vi "TestExecutive.vi"() -> ()   [LabVIEW 2025]
uses:
  controls/TestDefinition.ctl
  controls/TestType.ctl
  controls/TestExecStates.ctl
  <vilib>/Utility/error.llb/DialogType.ctl
  <vilib>/Utility/error.llb/Error Cluster From Error Code.vi
  <vilib>/ErrorRing/Error Ring.xnode
panel:
  out "Camera":string="USB Camera"
  out "TopFolderPath":path=path "E:/LTM Tests/HeaterTest_25-01-22_17-59-34"
  out "TopFolderPrefix":string="HeaterTest_25-01-22_17-59-34"
  in  "Server IP":u16(ring) items=["localhost", "172.17.52.10"]
  out "Status":string="Waiting for Rising trigger. Target = -50.000000"
  in  "Main Tabs":T1(tab)=enum."TestDefinition"
  in  "Next Button 2":bool
  in  "Loggers Directory":path=path "E:/LTM Tests/MechanismLTM"
  in  "Test Name":string="HeaterTest"
  in  "FFMPEG exe":path=path "C:/Program Files/FFMpeg/bin/ffmpeg.exe"
  in  "Path to Actuation Script":path=path "C:/Users/Public/Documents/ob_egse-ABU_LTM_MotorTesting/egse.py"
  in  "StartCycle":i32
  in  "Next Button":bool
  in  "PSU_Monitor":waveform(dbl)[](array[waveform])=[{"t0"=timestamp(3820413812.1099424 s since 1904-01-01), "dt"=1.0, "Y"=[2.52], "attributes"=variant("NI_ChannelName"=variant(string "Board_Voltage_0"))}, {"t0"=timestamp(3820413812.1153584 s since 1904-01-01), "dt"=1.0, "Y"=[-0.009], "attributes"=variant("NI_ChannelName"=variant(string "Board_Voltage_0"))}, {"t0"=timestamp(3820413812.1099424 s since 1904-01-01), "dt"=1.0, "Y"=[-0.017], "attributes"=variant("NI_ChannelName"=variant(string "Board_Current_0"))}, {"t0"=timestamp(3820413812.1153584 s since 1904-01-01), "dt"=1.0, "Y"=[0.0], "attributes"=variant("NI_ChannelName"=variant(string "Board_Current_0"))}]
  in  "Heater Monitor":waveform(dbl)[](array[waveform])=[{"t0"=timestamp(3820413812.092942 s since 1904-01-01), "dt"=1.0, "Y"=[-0.005], "attributes"=variant("NI_ChannelName"=variant(string "Heater_Voltage"))}, {"t0"=timestamp(3820413812.092942 s since 1904-01-01), "dt"=1.0, "Y"=[-0.002], "attributes"=variant("NI_ChannelName"=variant(string "Heater_Current"))}]
  in  "Video Camera":u16(ring) items=["USB Camera"]
  out "ChannelNames":string[](array[string])=["3A", "3B", "3C", "3D", "4A", "4B", "4C", "4D", "Target"]
  in  "ControlChannel":u16(ring) items=["3A", "3B", "3C", "3D", "4A", "4B", "4C", "4D", "Target"]
  in  "TVC_Temperatures":waveform(dbl)[](array[waveform])=[{"t0"=timestamp(3820413812.1049423 s since 1904-01-01), "dt"=1.0, "Y"=[-80.0], "attributes"=variant("NI_ChannelName"=variant(string "3A"))}, {"t0"=timestamp(3820413812.1049423 s since 1904-01-01), "dt"=1.0, "Y"=[0.1969585335155295], "attributes"=variant("NI_ChannelName"=variant(string "3B"))}, {"t0"=timestamp(3820413812.1049423 s since 1904-01-01), "dt"=1.0, "Y"=[0.2898606356704896], "attributes"=variant("NI_ChannelName"=variant(string "3C"))}, {"t0"=timestamp(3820413812.1049423 s since 1904-01-01), "dt"=1.0, "Y"=[0.3274623555028864], "attributes"=variant("NI_ChannelName"=variant(string "3D"))}, {"t0"=timestamp(3820413812.1049423 s since 1904-01-01), "dt"=1.0, "Y"=[0.3794250746071903], "attributes"=variant("NI_ChannelName"=variant(string "4A"))}, {"t0"=timestamp(3820413812.1049423 s since 1904-01-01), "dt"=1.0, "Y"=[0.7650917242886434], "attributes"=variant("NI_ChannelName"=variant(string "4B"))}, {"t0"=timestamp(3820413812.1049423 s since 1904-01-01), "dt"=1.0, "Y"=[0.4416685188806395], "attributes"=variant("NI_ChannelName"=variant(string "4C"))}, {"t0"=timestamp(3820413812.1049423 s since 1904-01-01), "dt"=1.0, "Y"=[0.7497510727682433], "attributes"=variant("NI_ChannelName"=variant(string "4D"))}, {"t0"=timestamp(3820413812.1049423 s since 1904-01-01), "dt"=1.0, "Y"=[0.8015992709050663], "attributes"=variant("NI_ChannelName"=variant(string "Target"))}]
  in  "TLUP_Temperatures":waveform(dbl)[](array[waveform])=[{"t0"=timestamp(3820413812.102944 s since 1904-01-01), "dt"=1.0, "Y"=[23.56152], "attributes"=variant("NI_ChannelName"=variant(string "TLUP_0"))}, {"t0"=timestamp(3820413812.102944 s since 1904-01-01), "dt"=1.0, "Y"=[-999.0], "attributes"=variant("NI_ChannelName"=variant(string "TLUP_1"))}, {"t0"=timestamp(3820413812.102944 s since 1904-01-01), "dt"=1.0, "Y"=[-999.0], "attributes"=variant("NI_ChannelName"=variant(string "TLUP_2"))}, {"t0"=timestamp(3820413812.102944 s since 1904-01-01), "dt"=1.0, "Y"=[-999.0], "attributes"=variant("NI_ChannelName"=variant(string "TLUP_3"))}, {"t0"=timestamp(3820413812.102944 s since 1904-01-01), "dt"=1.0, "Y"=[nan], "attributes"=variant("NI_ChannelName"=variant(string "TLUP_4"))}, {"t0"=timestamp(3820413812.102944 s since 1904-01-01), "dt"=1.0, "Y"=[nan], "attributes"=variant("NI_ChannelName"=variant(string "TLUP_5"))}, {"t0"=timestamp(3820413812.102944 s since 1904-01-01), "dt"=1.0, "Y"=[nan], "attributes"=variant("NI_ChannelName"=variant(string "TLUP_6"))}, {"t0"=timestamp(3820413812.102944 s since 1904-01-01), "dt"=1.0, "Y"=[nan], "attributes"=variant("NI_ChannelName"=variant(string "TLUP_7"))}]
  in  "PSU Enable":bool
  in  "Heater Enable":bool
  in  "COM Port":i32=21 min=1 max=63 step=1
  in  "TestDefinition":T2={"Tests"=[{"TTrigger"=-130.0, "Direction"=enum."Falling", "TDelay"=0.0, "Type"=enum."No Test", "Heater Test (s)"=0.0, "Pre-Log (s)"=0.0, "Post-Log(s)"=0.0}, {"TTrigger"=-80.0, "Direction"=enum."Rising", "TDelay"=0.0, "Type"=enum."Heater Test", "Heater Test (s)"=900.0, "Pre-Log (s)"=10.0, "Post-Log(s)"=100.0}, {"TTrigger"=-50.0, "Direction"=enum."Rising", "TDelay"=30.0, "Type"=enum."No Test", "Heater Test (s)"=0.0, "Pre-Log (s)"=0.0, "Post-Log(s)"=0.0}, {"TTrigger"=-50.0, "Direction"=enum."Rising", "TDelay"=0.0, "Type"=enum."Heater Test", "Heater Test (s)"=150.0, "Pre-Log (s)"=10.0, "Post-Log(s)"=0.0}, {"TTrigger"=-50.0, "Direction"=enum."Rising", "TDelay"=0.0, "Type"=enum."Actuation Test", "Heater Test (s)"=0.0, "Pre-Log (s)"=2.0, "Post-Log(s)"=10.0}, {"TTrigger"=-45.0, "Direction"=enum."Rising", "TDelay"=0.0, "Type"=enum."Actuation Test", "Heater Test (s)"=30.0, "Pre-Log (s)"=10.0, "Post-Log(s)"=100.0}, {"TTrigger"=-35.0, "Direction"=enum."Rising", "TDelay"=0.0, "Type"=enum."Actuation Test", "Heater Test (s)"=30.0, "Pre-Log (s)"=10.0, "Post-Log(s)"=100.0}, {"TTrigger"=-25.0, "Direction"=enum."Rising", "TDelay"=0.0, "Type"=enum."Actuation Test", "Heater Test (s)"=30.0, "Pre-Log (s)"=10.0, "Post-Log(s)"=100.0}, {"TTrigger"=-15.0, "Direction"=enum."Rising", "TDelay"=0.0, "Type"=enum."Actuation Test", "Heater Test (s)"=30.0, "Pre-Log (s)"=10.0, "Post-Log(s)"=100.0}, {"TTrigger"=0.0, "Direction"=enum."Rising", "TDelay"=0.0, "Type"=enum."Actuation Test", "Heater Test (s)"=30.0, "Pre-Log (s)"=10.0, "Post-Log(s)"=100.0}, {"TTrigger"=10.0, "Direction"=enum."Rising", "TDelay"=0.0, "Type"=enum."Actuation Test", "Heater Test (s)"=30.0, "Pre-Log (s)"=10.0, "Post-Log(s)"=100.0}, {"TTrigger"=30.0, "Direction"=enum."Rising", "TDelay"=0.0, "Type"=enum."Actuation Test", "Heater Test (s)"=30.0, "Pre-Log (s)"=10.0, "Post-Log(s)"=100.0}, {"TTrigger"=40.0, "Direction"=enum."Rising", "TDelay"=0.0, "Type"=enum."Actuation Test", "Heater Test (s)"=30.0, "Pre-Log (s)"=10.0, "Post-Log(s)"=100.0}, {"TTrigger"=40.0, "Direction"=enum."Rising", "TDelay"=30.0, "Type"=enum."No Test", "Heater Test (s)"=30.0, "Pre-Log (s)"=10.0, "Post-Log(s)"=100.0}], "ActuationsPerLoop"=2, "Temperature\nLog Period(ms)"=1000, "PSU \nLog Period (ms)"=100} {"Tests"."Post-Log(s)" format="%#_13g"; "Tests"."Pre-Log (s)" format="%#_13g"; "Tests"."Heater Test (s)" format="%#_13g"}
  in  "Next Button 3":bool
  out "Master Logging":bool=TRUE
  out "DelayRemaining":string="00:00"
  out "Heater On":bool
  out "Temperatures":dynamicdata(graph)
  out "Trigger Point Reading":dbl=-80.0
  out "Actuation Logging":bool
  out "Heater Logging":bool
  in  "CyclesRemaining":i32
  in  "TempCycleNo":i32
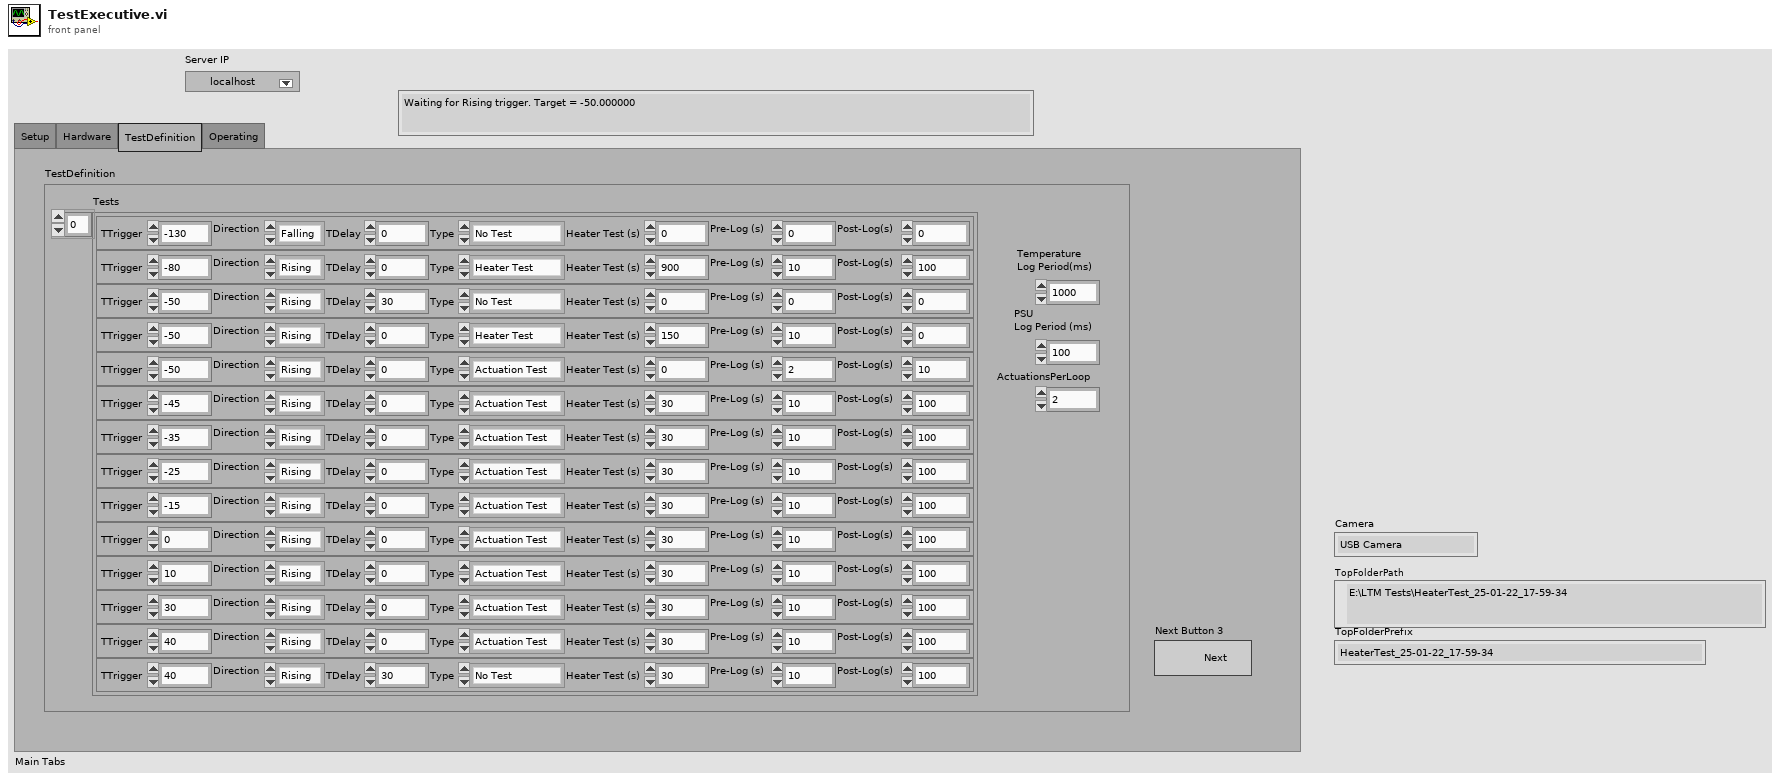
[diagram p1: front panel]
types:
  T1 = enum32{"Setup", "Hardware", "TestDefinition", "Operating"}
  T2 = typedef "TestDefinition.ctl" = cluster{"Tests":cluster{"TTrigger":dbl, "Direction":enum16{"Rising", "Falling"}, "TDelay":dbl, "Type":T3, "Heater Test (s)":dbl, "Pre-Log (s)":dbl, "Post-Log(s)":dbl}[], "ActuationsPerLoop":i32, "Temperature\nLog Period(ms)":i64, "PSU \nLog Period (ms)":i64}
  T3 = typedef "TestType.ctl" = enum16{"No Test", "Heater Test", "Actuation Test"}
  T4 = typedef "TestExecStates.ctl" = enum16{"Initialise", "Check Inputs", "Check Hardware", "Review Tests", "RunTests", "AbortExit", "Shutdown"}
  T5 = enum32{"Invalid Status", "Unconnected", "Active", "Idle", "Error", "Connecting"}
  T6 = typedef "LVDataSocketStatusTypeDef.ctl" = cluster{"Code":enum32{"Invalid Status", "Unconnected", "Active", "Idle", "Error", "Connecting"}, "Text":string}
  T7 = typedef "DialogType.ctl" = u16
  T8 = cluster{"TTrigger":dbl, "Direction":enum16{"Rising", "Falling"}, "TDelay":dbl, "Type":T3, "Heater Test (s)":dbl, "Pre-Log (s)":dbl, "Post-Log(s)":dbl}[]
  T9 = typedef "FFMpegRef.ctl" = cluster{"FFMpegRef":refnum<k24>, "StdOutRef":refnum<k24>, "DiagRef":refnum<k24>}
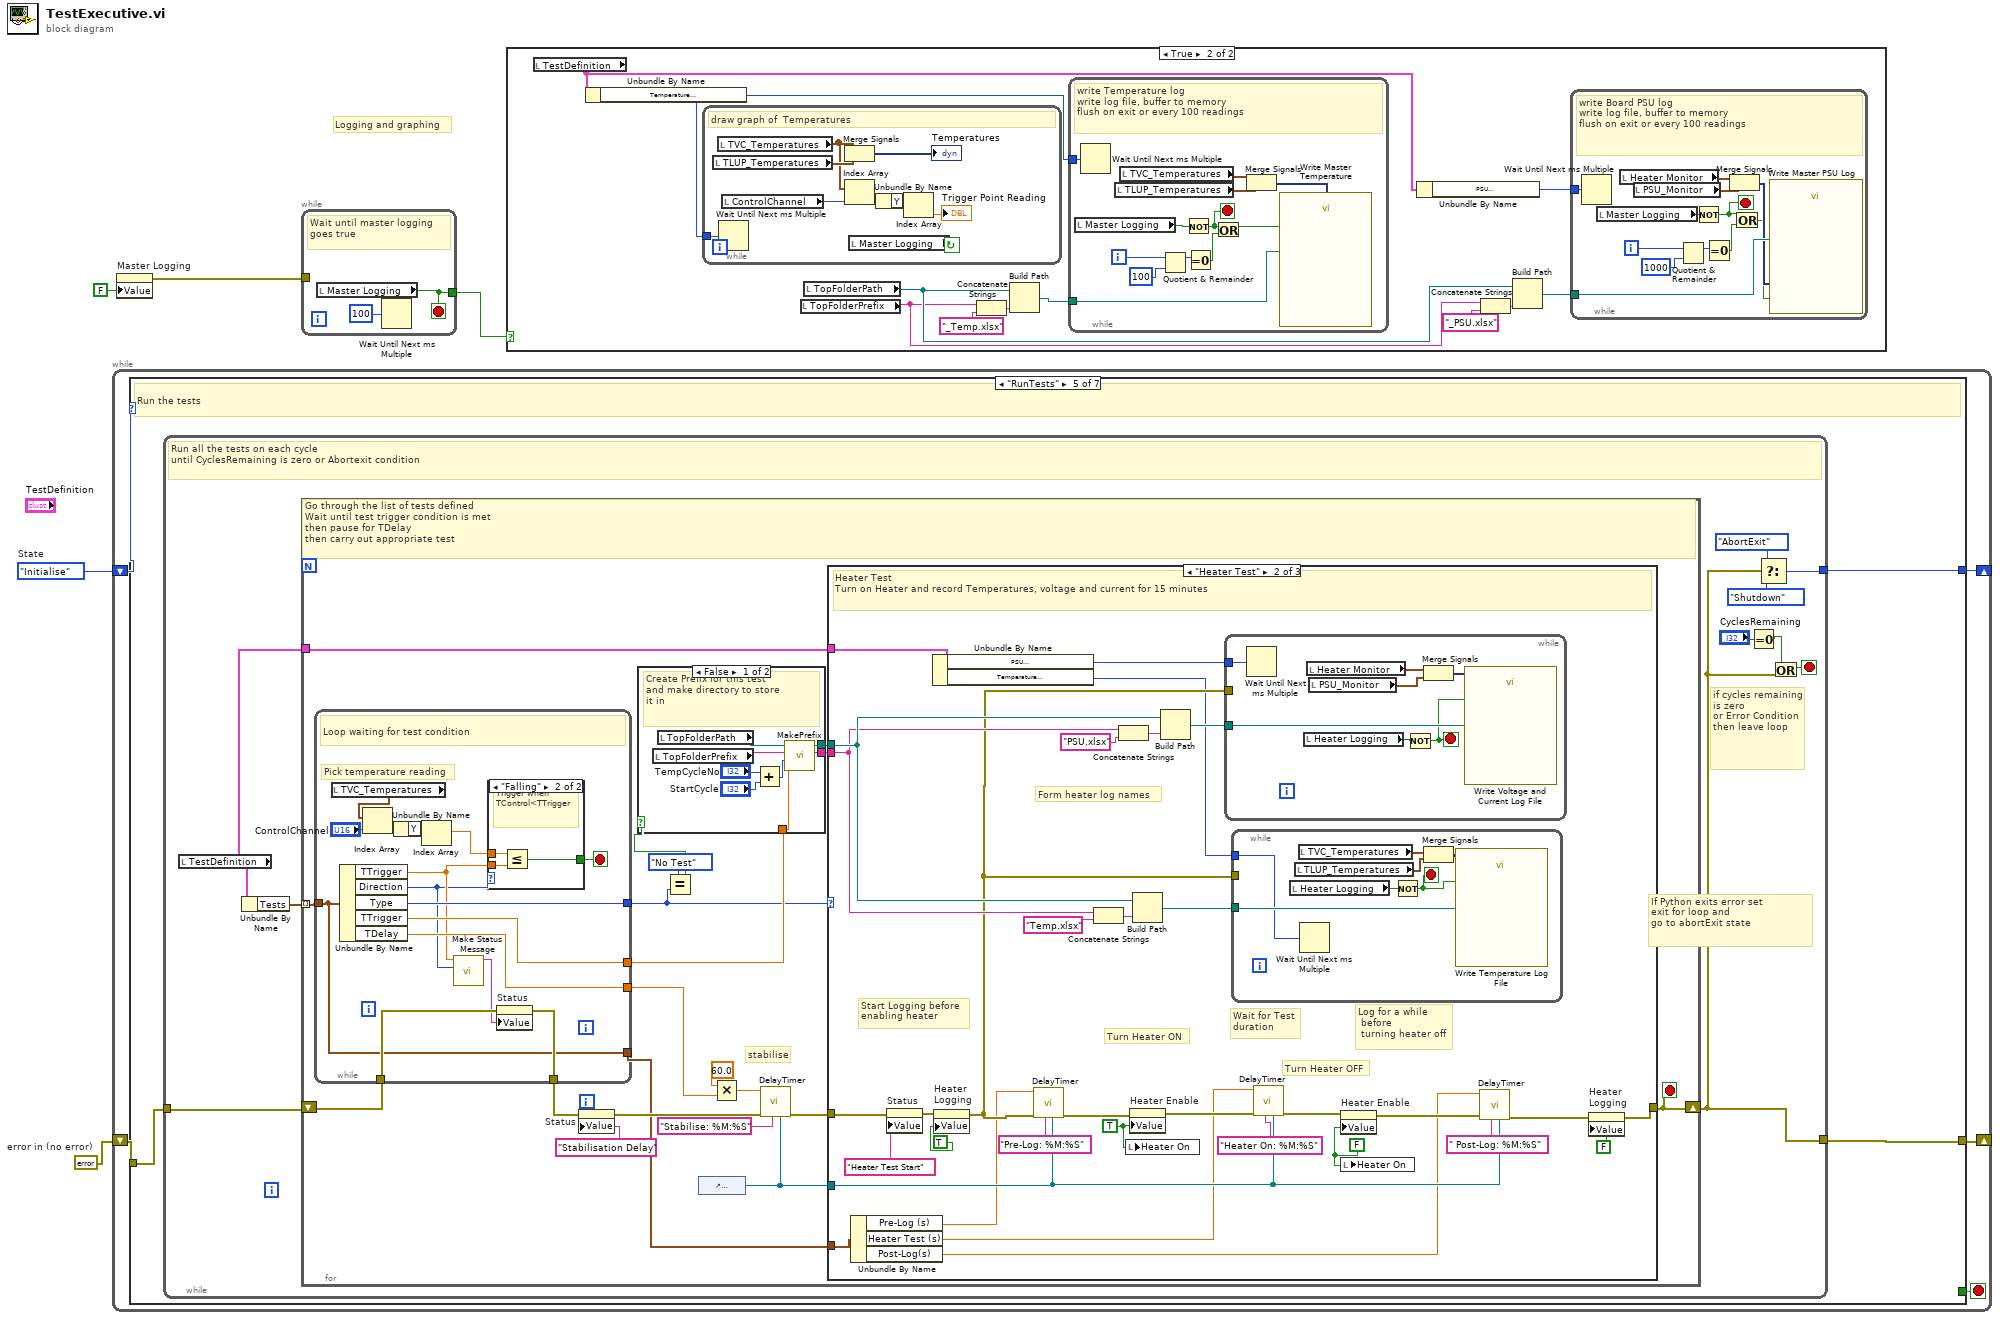
[diagram p0: block diagram]
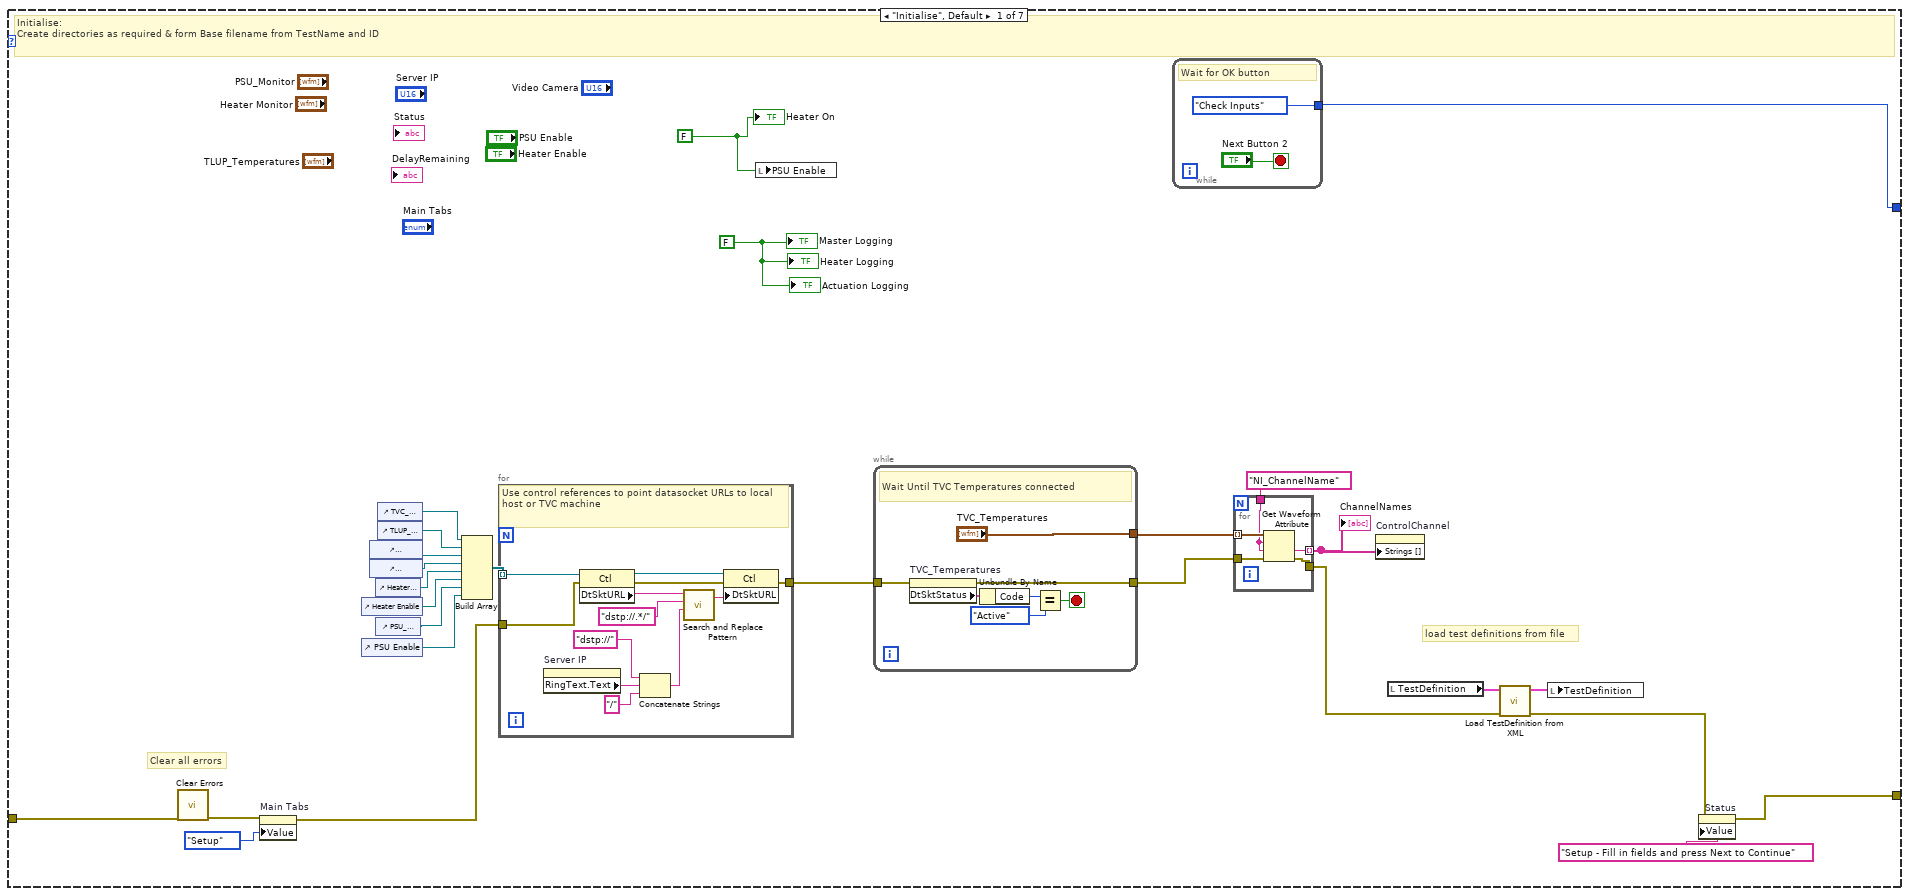
[diagram p3: hidden frame]
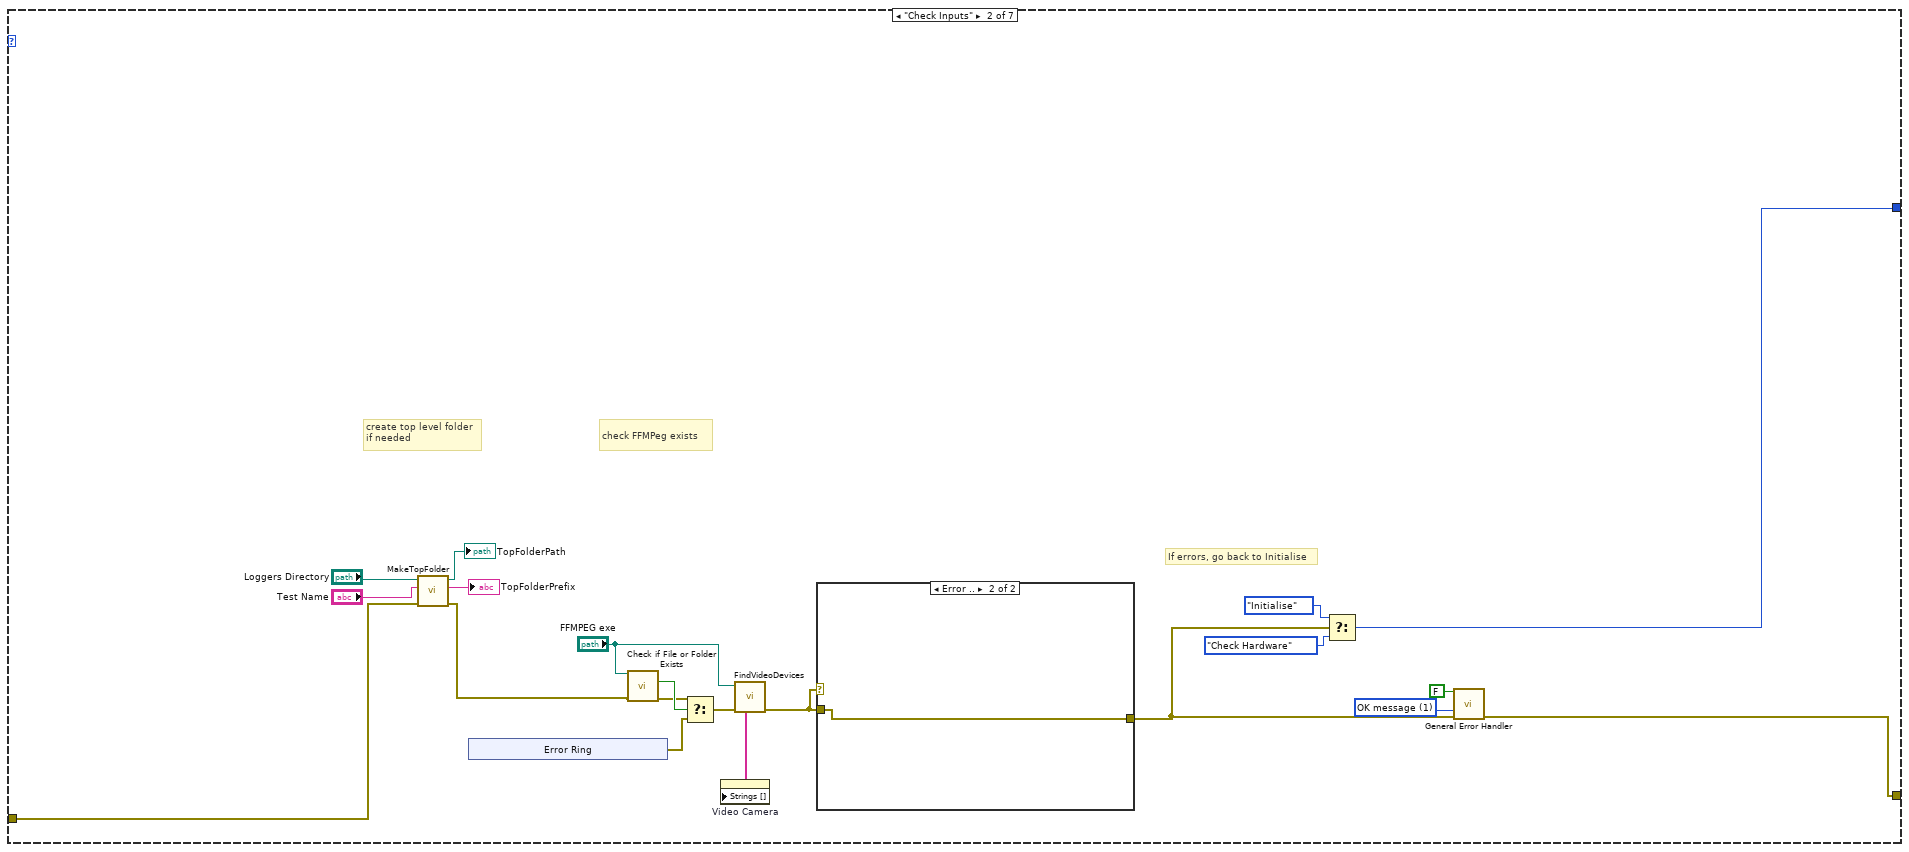
[diagram p4: hidden frame]
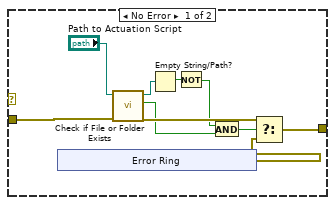
[diagram p5: hidden frame]
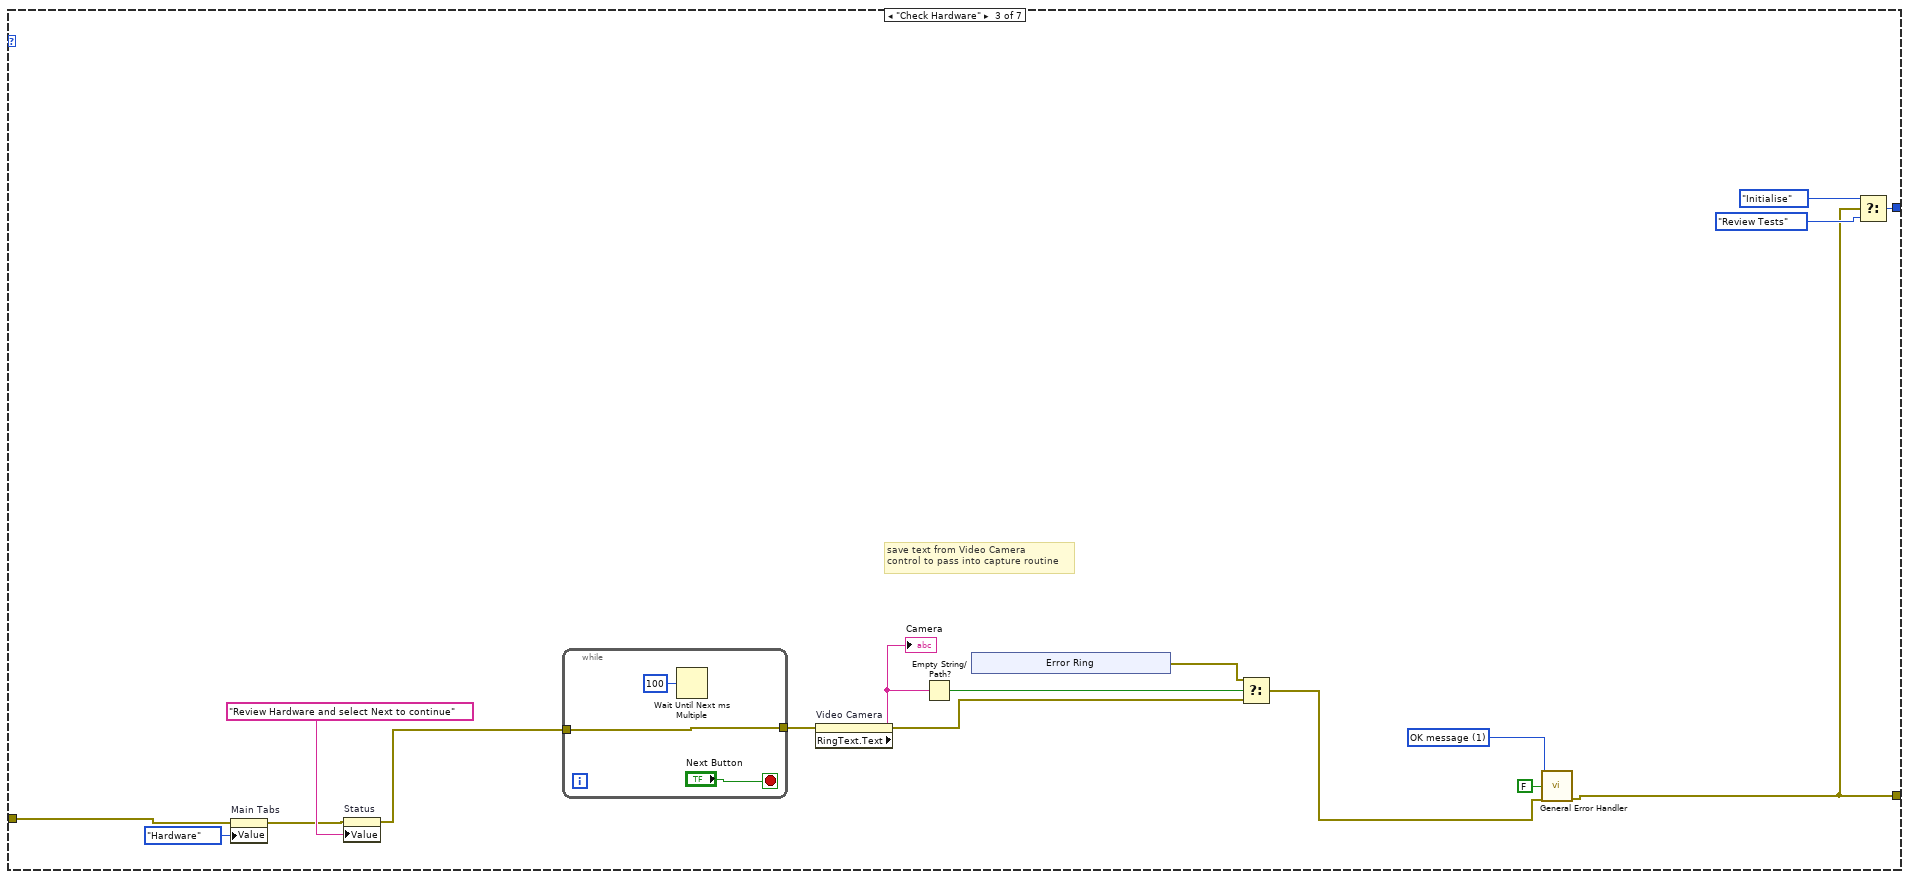
[diagram p6: hidden frame]
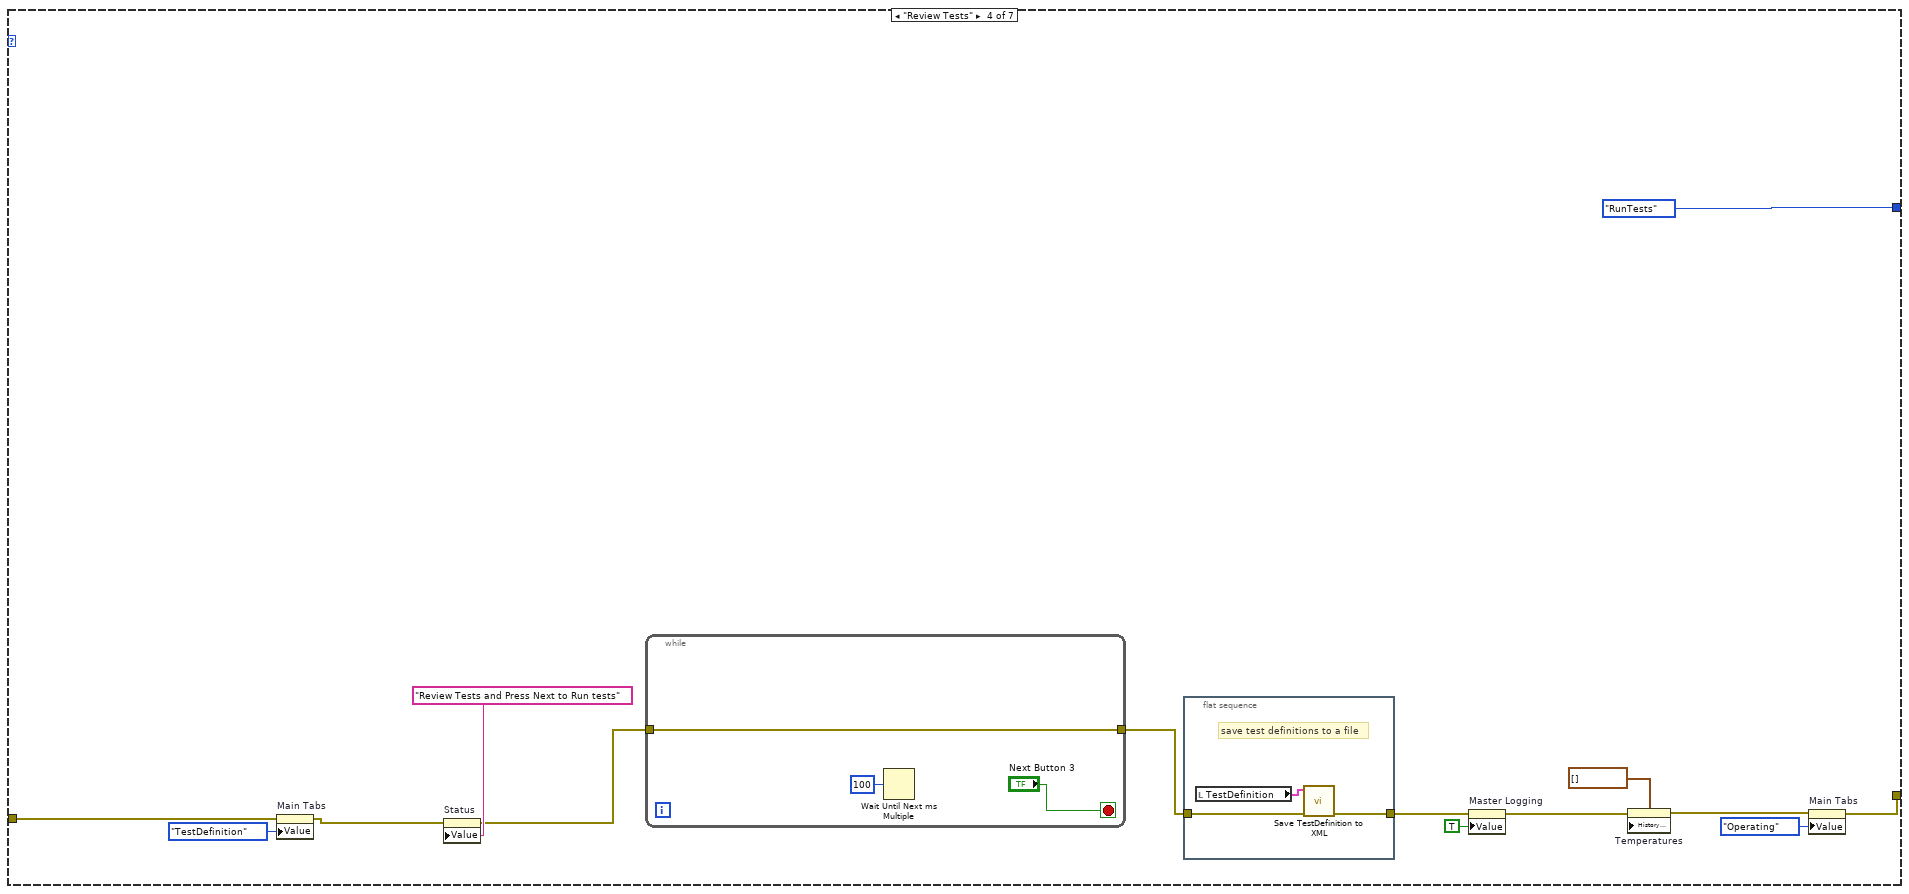
[diagram p7: hidden frame]
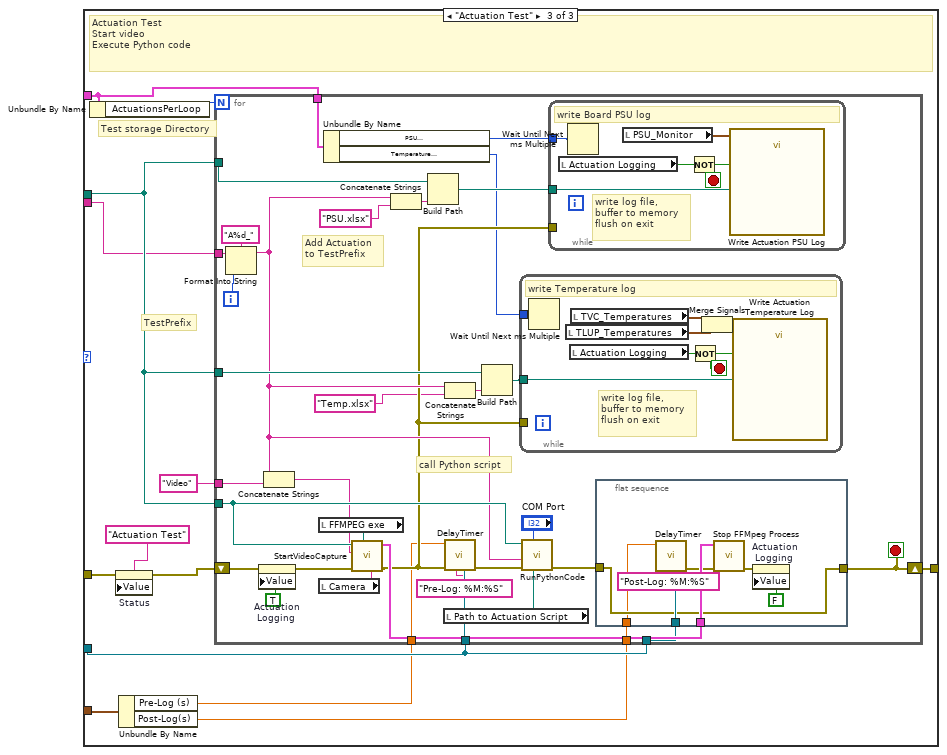
[diagram p10: hidden frame]
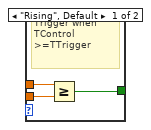
[diagram p11: hidden frame]
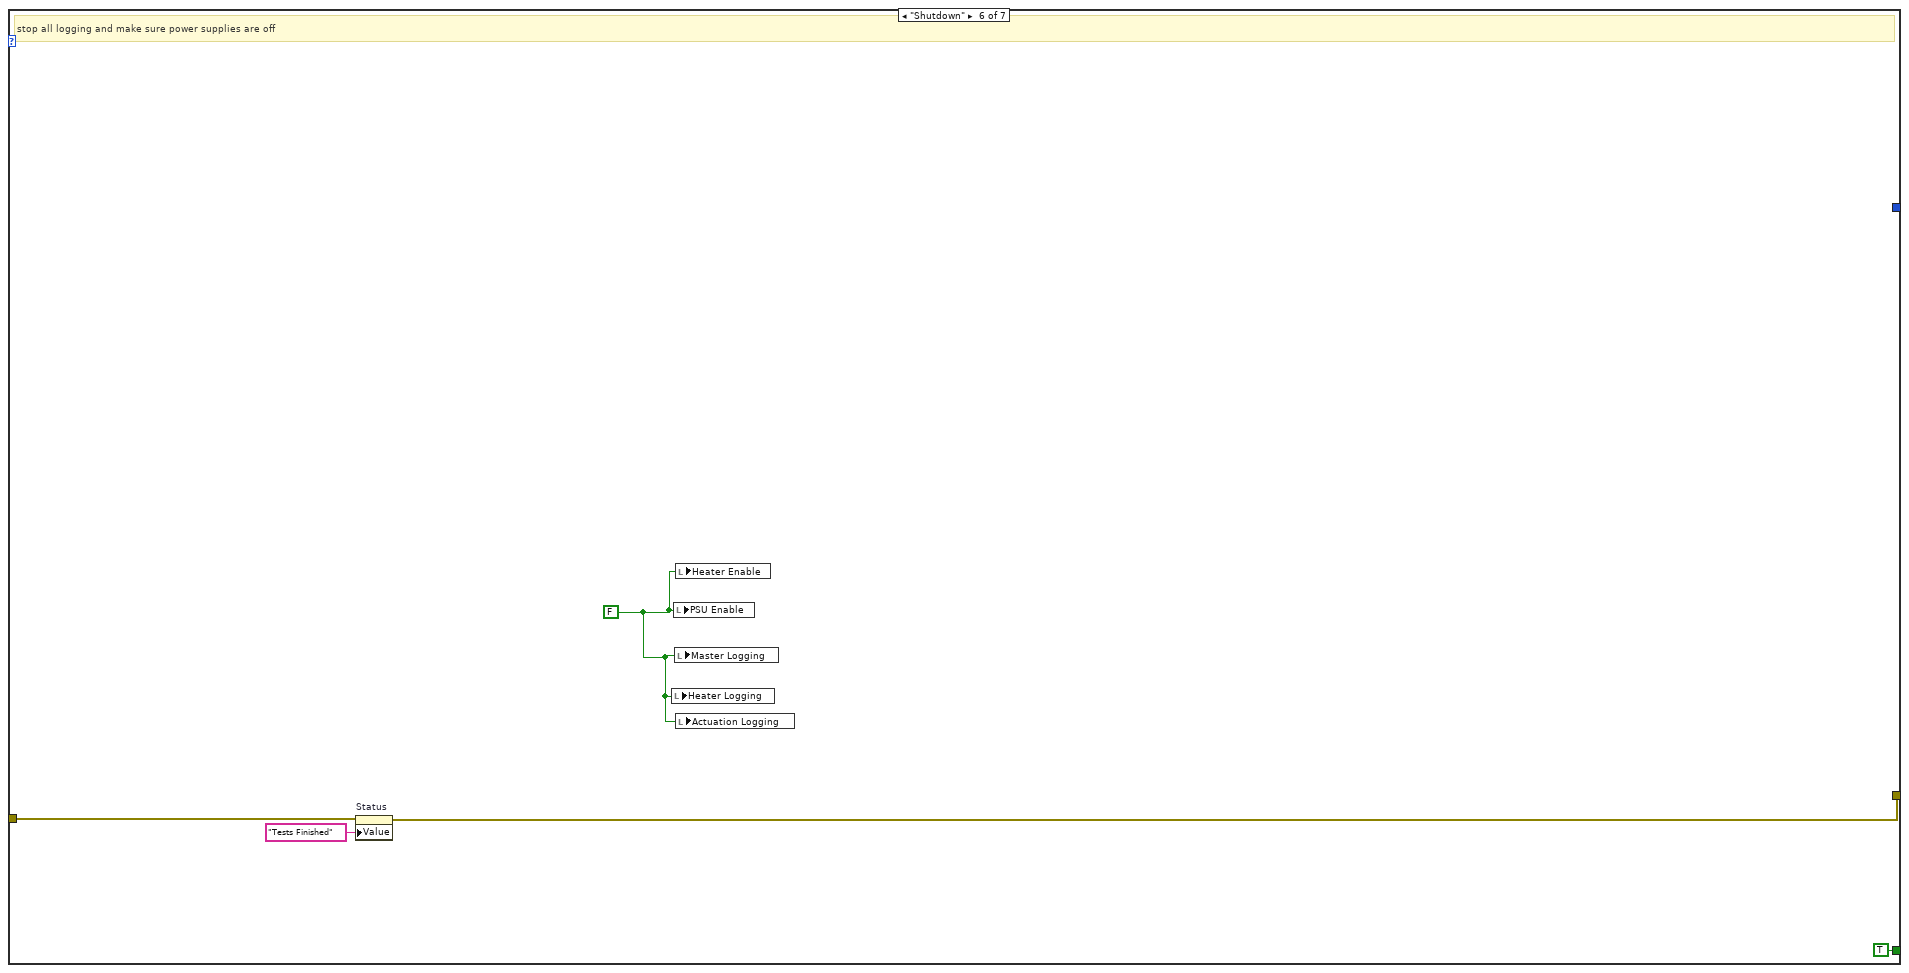
[diagram p12: hidden frame]
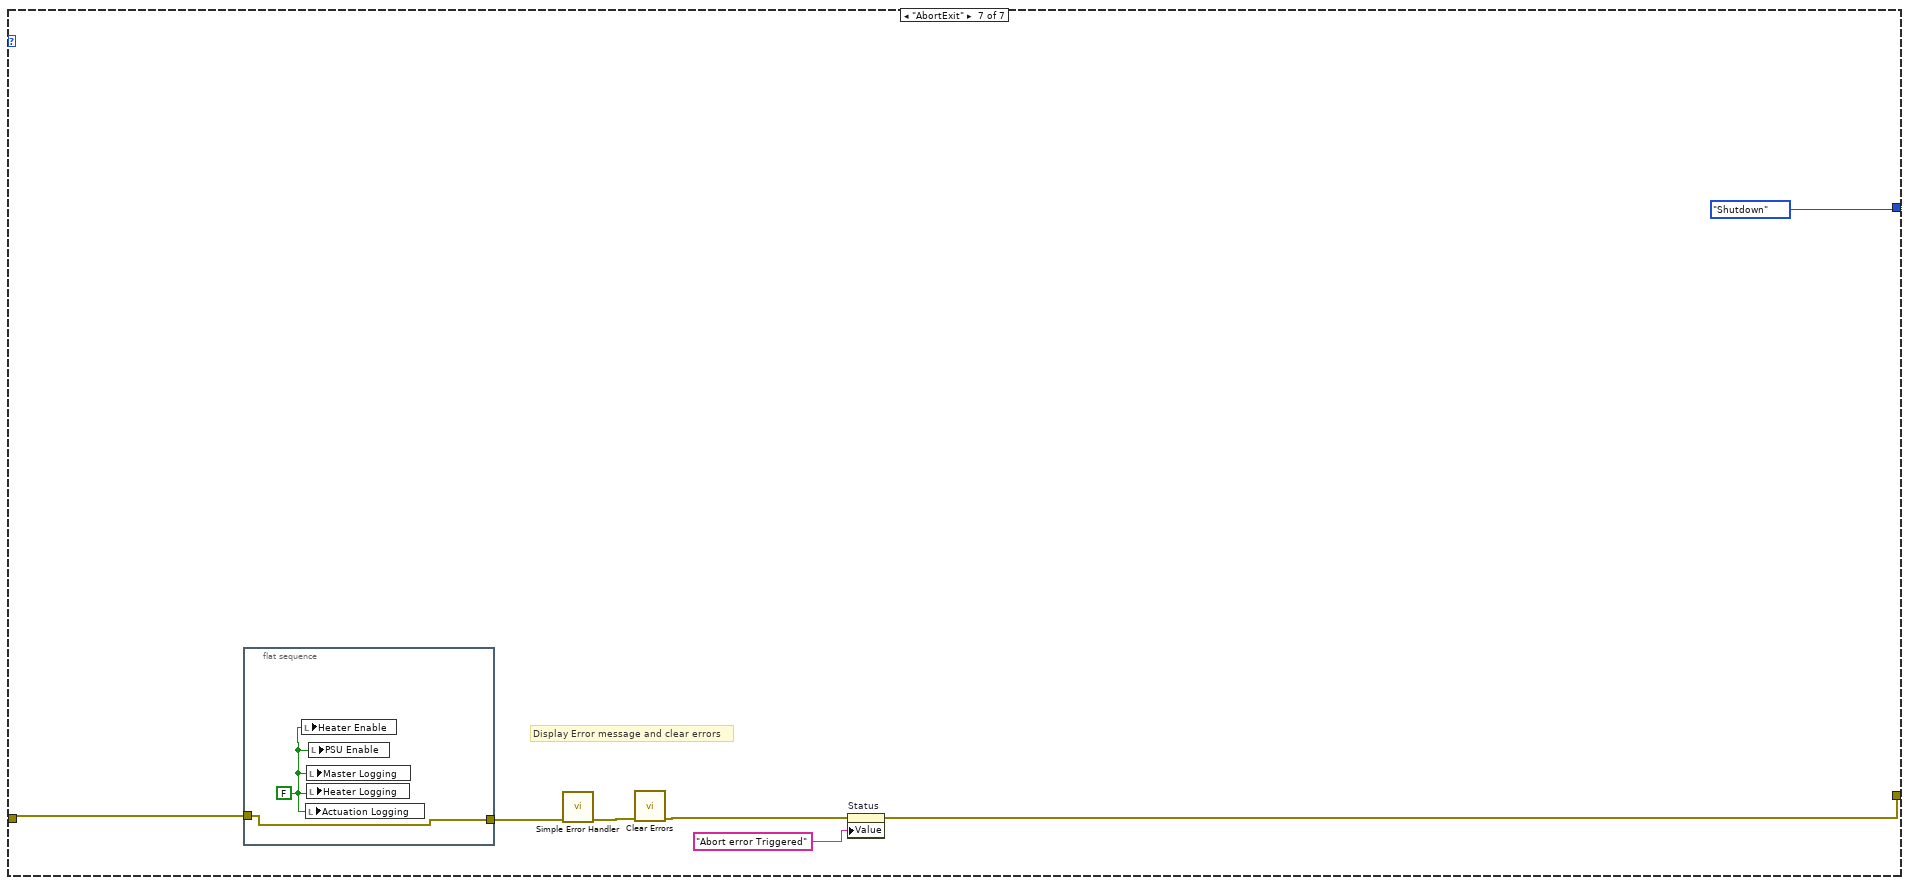
[diagram p13: hidden frame]
diagram:
  w4 = errorcluster {"status"=FALSE, "code"=0, "source"=""}  # error in (no error)
  w5 = TestExecStates."Initialise"  # State
  # "Logging and graphing"
  n1 = while {
    shift-right: [w9] -> _
    shift-left: w5 -> [w10]
    shift-right: [w8] -> _
    shift-left: w4 -> [w7]
    stop <- w6 stop-if-true
    n2 = case shown="\"RunTests\"" w10 {
      tunnel: [w22 w66 w107 TestExecStates."RunTests" ("State") w147 _ TestExecStates."Shutdown" ("State")] -> w9
      tunnel: [w23 w77 w104 w134 w148 w327 w335] -> w8
      tunnel: w7 -> [w19 w79 w118 w137 w149 w328 w331]
      tunnel: [_ _ _ _ _ TRUE _] -> w6
      frame "Initialise", Default {
        w17 = FALSE ("Heater Enable")
        w18 = FALSE ("Master Logging")
        # "load test definitions from file"
        # "Clear all errors"
        # "Initialise:\nCreate directories as required & form Base filename from TestName and ID"
        n3 = call <vilib>:"Clear Errors.vi"("error in (no error)"=w19) -> ("error out"=w16:errorcluster)  [unwired: 5 in, 1 out]
        n4 = property on="Main Tabs" class="TabCtl (strict)"(error in=w16, "Value"=T1."Setup" ("Main Tabs")) -> (error out=w15:errorcluster)  [unwired: 1 in, 1 out]
        n5 = control-ref of="Heater Enable"() -> (w29:refnum<vi>)
        n6 = control-ref of="PSU Enable"() -> (w30:refnum<vi>)
        n7 = control-ref of="CyclesRemaining"() -> (w28:refnum<vi>)
        n8 = control-ref of="TempCycleNo"() -> (w32:refnum<vi>)
        n9 = control-ref of="Heater Monitor"() -> (w25:refnum<vi>)
        n10 = control-ref of="PSU_Monitor"() -> (w24:refnum<vi>)
        n11 = control-ref of="TVC_Temperatures"() -> (w27:refnum<vi>)
        n12 = control-ref of="TLUP_Temperatures"() -> (w31:refnum<vi>)
        n13 = Build Array(w27, w31, w28, w32, w25, w29, w24, w30) -> (w26:refnum<vi>[])
        n14 = for {
          tunnel: w26 -> [w49] mode=indexing
          tunnel: [w40] -> w33
          tunnel: w15 -> [w38]
          # "Use control references to point datasocket URLs to local host or TVC machine"
          n15 = property on="Server IP" class="Ring (strict)"() -> ("RingText.Text"=w48:string)  [unwired: 2 in, 2 out]
          n16 = property class="Ctl"(reference=w49, error in=w38) -> (reference out=w42:refnum<vi>, error out=w39:errorcluster, "DtSktURL"=w45:string)
          n17 = Concatenate Strings("dstp://" ("string"), w48, "/" ("string")) -> (w44:string)
          n18 = call <vilib>:"Search and Replace Pattern.vi"("string"=w45, "regular expression (\"\")"="dstp://.*/" ("regular expression (\"\")"), "replace string (\"\")"=w44) -> ("result string"=w41:string)  [unwired: 2 in, 1 out]
          n19 = property class="Ctl"(reference=w42, error in=w39, "DtSktURL"=w41) -> (error out=w40:errorcluster)  [unwired: 1 out]
        }
        n20 = local write "PSU Enable"(w17) -> ()
        n21 = while {
          tunnel: ["TVC_Temperatures"] -> w36
          tunnel: w33 -> [w56]
          tunnel: [w55] -> w21
          stop <- w58 stop-if-true
          # "Wait Until TVC Temperatures connected"
          n22 = property on="TVC_Temperatures" class="Arr (strict)"(error in=w56) -> (error out=w55:errorcluster, "DtSktStatus"=w61:T6)  [unwired: 1 in, 1 out]
          n23 = Unbundle By Name(w61) -> ("Code"=w60:T5)
          n24 = Equal?(x=w60, y=T5."Active") -> (x = y?=w58:bool)
        }
        n25 = while {
          tunnel: [TestExecStates."Check Inputs" ("State")] -> w22
          stop <- "Next Button 2" stop-if-true
          # "Wait for OK button"
        }
        n26 = for {
          tunnel: w36 -> [w54] mode=indexing
          tunnel: "NI_ChannelName" ("name") -> [w53]
          tunnel: [w52] -> w34 mode=indexing
          tunnel: w21 -> [w51]
          tunnel: [w50] -> w20
          n27 = Get Waveform Attribute(4:w51, 5:w53, 6:w53, 7:w54) -> (0:w50:errorcluster, 1:w52:string)  [unwired: 2 out]
        }
        "ChannelNames" <- w34
        n28 = property on="ControlChannel" class="Ring (strict)"("Strings []"=w34) -> ()  [unwired: 2 in, 2 out]
        n29 = local read "TestDefinition"() -> (w12:T2)
        n30 = call "Load TestDefinition from XML.vi"("error in (no error)"=w20, "TestDefinition"=w12) -> ("error out"=w13:errorcluster, "User Specified Out"=w11:T2)  [unwired: 8 in]
        n31 = local write "TestDefinition"(w11) -> ()
        n32 = property on="Status" class="Str"(error in=w13, "Value"="Setup - Fill in fields and press Next to Continue" ("Status")) -> (error out=w23:errorcluster)  [unwired: 1 in, 1 out]
        "Master Logging" <- w18
        "Heater On" <- w17
        "Heater Logging" <- w18
        "Actuation Logging" <- w18
      }
      frame "Check Inputs" {
        w78 = T7 1 items=["no dialog", "OK message", "continue or stop message", "OK message + warnings", "continue/stop + warnings"] ("type of dialog (OK msg:1)")
        # "If errors, go back to Initialise"
        # "create top level folder\nif needed"
        # "check FFMPeg exists"
        n33 = call "MakeTopFolder.vi"("error in (no error)"=w79, "Comment"="Test Name", "Loggers"="Loggers Directory") -> ("error out"=w75:errorcluster, "TopFolderPrefix"=→"TopFolderPrefix":string, "TestFolderPath"=→"TopFolderPath":path)  [unwired: 6 in]
        n34 = xnode "Error Ring"() -> ("error out"=w72:errorcluster)
        n35 = call <vilib>:"Check if File or Folder Exists.vi"("error in (no error)"=w75, "path"="FFMPEG exe") -> ("error out"=w73:errorcluster, "file or folder exists?"=w74:bool)  [unwired: 7 in, 1 out]
        n36 = Select(t=w73, s=w74, f=w72) -> (s? t:f=w71:errorcluster)
        n37 = call "FindVideoDevices.vi"("error in (no error)"=w71, "Path to FFMPEG"="FFMPEG exe") -> ("error out"=w65:errorcluster, "Video Devices"=w76:string[])  [unwired: 8 in]
        n38 = property on="Video Camera" class="Ring (strict)"("Strings []"=w76) -> ()  [unwired: 2 in, 2 out]
        n39 = case shown="Error .." w65 {
          tunnel: w65 -> [w90 w98]
          tunnel: [w89 w98] -> w69
          frame No Error {
            n40 = xnode "Error Ring"() -> ("error out"=w91:errorcluster)
            n41 = call <vilib>:"Check if File or Folder Exists.vi"("error in (no error)"=w90, "path"="Path to Actuation Script") -> ("error out"=w92:errorcluster, "file or folder exists?"=w84:bool, "dup path"=w88:path)  [unwired: 7 in]
            n42 = Empty String/Path?(string/path=w88) -> (empty?=w86:bool)
            n43 = Not(x=w86) -> (.not. x?=w85:bool)
            n44 = And(x=w85, y=w84) -> (x .and. y?=w87:bool)
            n45 = Select(t=w92, s=w87, f=w91) -> (s? t:f=w89:errorcluster)
          }
          frame Error {
          }
        }
        n46 = Select(t=TestExecStates."Initialise" ("State"), s=w69, f=TestExecStates."Check Hardware" ("State")) -> (s? t:f=w66:T4)
        n47 = call <vilib>:"General Error Handler.vi"("search ni.com link visible?(T)"=FALSE, "type of dialog (OK msg:1)"=w78, "error in (no error)"=w69) -> ("error out"=w77:errorcluster)  [unwired: 8 in, 4 out]
      }
      frame "Check Hardware" {
        w109 = T7 1 items=["no dialog", "OK message", "continue or stop message", "OK message + warnings", "continue/stop + warnings"] ("type of dialog (OK msg:1)")
        # "save text from Video Camera \ncontrol to pass into capture routine"
        n48 = property on="Main Tabs" class="TabCtl (strict)"(error in=w118, "Value"=T1."Hardware" ("Main Tabs")) -> (error out=w117:errorcluster)  [unwired: 1 in, 1 out]
        n49 = property on="Status" class="Str"(error in=w117, "Value"="Review Hardware and select Next to continue" ("Status")) -> (error out=w115:errorcluster)  [unwired: 1 in, 1 out]
        n50 = while {
          tunnel: w115 -> [w125]
          tunnel: [w125] -> w114
          stop <- "Next Button" stop-if-true
          n51 = Wait Until Next ms Multiple(millisecond multiple=u32 100) -> ()  [unwired: 1 out]
        }
        n52 = property on="Video Camera" class="Ring (strict)"(error in=w114) -> (error out=w111:errorcluster, "RingText.Text"=w113:string)  [unwired: 1 in, 1 out]
        "Camera" <- w113
        n53 = Empty String/Path?(string/path=w113) -> (empty?=w112:bool)
        n54 = xnode "Error Ring"() -> ("error out"=w110:errorcluster)
        n55 = Select(t=w110, s=w112, f=w111) -> (s? t:f=w108:errorcluster)
        n56 = call <vilib>:"General Error Handler.vi"("search ni.com link visible?(T)"=FALSE, "type of dialog (OK msg:1)"=w109, "error in (no error)"=w108) -> ("error out"=w104:errorcluster)  [unwired: 8 in, 4 out]
        n57 = Select(t=TestExecStates."Initialise", s=w104, f=TestExecStates."Review Tests" ("State")) -> (s? t:f=w107:T4)
      }
      frame "Review Tests" {
        n58 = property on="Main Tabs" class="TabCtl (strict)"(error in=w137, "Value"=T1."TestDefinition" ("Main Tabs")) -> (error out=w138:errorcluster)  [unwired: 1 in, 1 out]
        n59 = property on="Status" class="Str"(error in=w138, "Value"="Review Tests and Press Next to Run tests" ("Status")) -> (error out=w135:errorcluster)  [unwired: 1 in, 1 out]
        n60 = while {
          tunnel: w135 -> [w144]
          tunnel: [w144] -> w130
          stop <- "Next Button 3" stop-if-true
          n61 = Wait Until Next ms Multiple(millisecond multiple=u32 100) -> ()  [unwired: 1 out]
        }
        n62 = flat-sequence {
          tunnel: w130 -> [w143]
          tunnel: [w142] -> w127
          frame #0 {
            # "save test definitions to a file"
            n63 = local read "TestDefinition"() -> (w141:T2)
            n64 = call "Save TestDefinition to XML.vi"("error in (no error)"=w143, "TestDefinition"=w141) -> ("error out"=w142:errorcluster)  [unwired: 9 in]
          }
        }
        n65 = property on="Master Logging" class="Bool (strict)"(error in=w127, "Value"=TRUE ("Graphing")) -> (error out=w131:errorcluster)  [unwired: 1 in, 1 out]
        n66 = property on="Temperatures" class="WFChart (strict)"(error in=w131, "History Data"=waveform(dbl)[] []) -> (error out=w132:errorcluster)  [unwired: 1 in, 1 out]
        n67 = property on="Main Tabs" class="TabCtl (strict)"(error in=w132, "Value"=T1."Operating" ("Main Tabs")) -> (error out=w134:errorcluster)  [unwired: 1 in, 1 out]
      }
      frame "RunTests" {
        # "Run the tests"
        n68 = while {
          tunnel: [w152] -> w148
          tunnel: w149 -> [w153]
          tunnel: [w154] -> w147
          stop <- w157 stop-if-true
          # "If Python exits error set\nexit for loop and \ngo to abortExit state"
          # "if cycles remaining is zero\nor Error Condition\nthen leave loop"
          # "Run all the tests on each cycle\nuntil CyclesRemaining is zero or Abortexit condition"
          n69 = local read "TestDefinition"() -> (w150:T2)
          n70 = Unbundle By Name(w150) -> ("Tests"=w151:T8)
          n71 = for {
            tunnel: w151 -> [w179] mode=indexing
            shift-right: [w166] -> w152
            shift-left: w153 -> [w172]
            tunnel: w150 -> [w161]
            stop <- w166 stop-if-true
            # "stabilise"
            # "Go through the list of tests defined \nWait until test trigger condition is met\nthen pause for TDelay\nthen carry out appropriate test"
            n72 = while {
              tunnel: w179 -> [w304]
              tunnel: [w314] -> w165
              tunnel: [w313] -> w175
              tunnel: [w312] -> w170
              tunnel: w172 -> [w309]
              tunnel: [w308] -> w171
              tunnel: [w304] -> w160
              stop <- w318 stop-if-true
              # "Pick temperature reading"
              # "Loop waiting for test condition"
              n73 = local read "TVC_Temperatures"() -> (w305:waveform(dbl)[])
              n74 = Unbundle By Name(w304) -> ("TTrigger"=w311:dbl, "Direction"=w310:enum16{"Rising", "Falling"}, "Type"=w314:T3, "TTrigger"=w312:dbl, "TDelay"=w313:dbl)
              n75 = Index Array(array=w305, index="ControlChannel") -> (element=w317:waveform(dbl))
              n76 = Unbundle By Name(w317) -> ("Y"=w315:dbl[])
              n77 = Index Array(array=w315) -> (element=w306:dbl)  [unwired: 1 in]
              n78 = call "Make Status Message.vi"("Direction"=w310, "TTrigger"=w311) -> ("Status Message"=w307:string)  [unwired: 9 in]
              n79 = case shown="\"Falling\"" w310 {
                tunnel: w306 -> [w320 w323]
                tunnel: w311 -> [w321 w324]
                tunnel: [w319 w322] -> w318
                frame "Rising", Default {
                  # "Trigger when TControl\n>=TTrigger"
                  n80 = Greater Or Equal?(x=w320, y=w321) -> (x >= y?=w319:bool)
                }
                frame "Falling" {
                  # "Trigger when TControl<TTrigger"
                  n81 = Less Or Equal?(x=w323, y=w324) -> (x <= y?=w322:bool)
                }
              }
              n82 = property on="Status" class="Str"(error in=w309, "Value"=w307) -> (error out=w308:errorcluster)  [unwired: 1 in, 1 out]
            }
            n83 = property on="Status" class="Str"(error in=w171, "Value"="Stabilisation Delay" ("Status")) -> (error out=w173:errorcluster)  [unwired: 1 in, 1 out]
            n84 = Equal?(x=TestType."No Test", y=w165) -> (x = y?=w163:bool)
            n85 = case shown="False" w163 {
              tunnel: w170 -> [w186 _]
              tunnel: [w185 _] -> w169
              tunnel: [w184 _] -> w168
              frame False {
                # "Create Prefix for this test\nand make directory to store \nit in"
                n86 = local read "TopFolderPrefix"() -> (w187:string)
                n87 = local read "TopFolderPath"() -> (w183:path)
                n88 = Add(x="TempCycleNo", y="StartCycle") -> (x+y=w180:i32)
                n89 = call "MakePrefix.vi"("TempPoint"=w186, "TempCycleNo"=w180, "FolderPrefix"=w187, "TopFolderPath"=w183) -> ("Prefix"=w184:string, "TestFolderPath"=w185:path)  [unwired: 6 in]
              }
              frame True {
                # "Don't create directory for null test"
              }
            }
            n90 = control-ref of="DelayRemaining"() -> (w167:refnum<vi>)
            n91 = Multiply(x=60.0 ("y"), y=w175) -> (x*y=w177:dbl)
            n92 = call "DelayTimer.vi"("Formatted \nTime Ref"=w167, "FormatString"="Stabilise: %M:%S", "error in (no error)"=w173, "Delay(s)"=w177) -> ("error out"=w176:errorcluster)  [unwired: 7 in]
            n93 = case shown="\"Heater Test\"" w165 {
              tunnel: w176 -> [w188 w210 w248]
              tunnel: [w188 w217 w246] -> w166
              tunnel: w169 -> [_ w204 w245]
              tunnel: w168 -> [_ w203 w242]
              tunnel: w167 -> [_ w197 w241]
              tunnel: w161 -> [_ w195 w236]
              tunnel: w160 -> [_ w192 w239]
              frame "No Test", Default {
                # "NoTest\nExit immediately and go to next test\nServes to wait for starting temperature to be reached"
              }
              frame "Heater Test" {
                w200 = TRUE ("Heater Logging")
                w201 = FALSE ("Heater PSU")
                # "Log for a while\n before\n turning heater off"
                # "Wait for Test \nduration"
                # "Turn Heater OFF"
                # "Turn Heater ON"
                # "Form heater log names"
                # "Start Logging before \nenabling heater"
                # "Heater Test\nTurn on Heater and record Temperatures, voltage and current for 15 minutes"
                n94 = Unbundle By Name(w192) -> ("Pre-Log (s)"=w191:dbl, "Heater Test (s)"=w190:dbl, "Post-Log(s)"=w189:dbl)
                n95 = property on="Status" class="Str"(error in=w210, "Value"="Heater Test Start" ("Status")) -> (error out=w209:errorcluster)  [unwired: 1 in, 1 out]
                n96 = Unbundle By Name(w195) -> ("PSU \nLog Period (ms)"=w194:i64, "Temperature\nLog Period(ms)"=w193:i64)
                n97 = property on="Heater\nLogging" class="Bool (strict)"(error in=w209, "Value"=TRUE ("Heater PSU")) -> (error out=w202:errorcluster)  [unwired: 1 in, 1 out]
                n98 = call "DelayTimer.vi"("Formatted \nTime Ref"=w197, "FormatString"="Pre-Log: %M:%S", "error in (no error)"=w202, "Delay(s)"=w191) -> ("error out"=w208:errorcluster)  [unwired: 7 in]
                n99 = Concatenate Strings(w203, "Temp.xlsx" ("string")) -> (w215:string)
                n100 = Concatenate Strings(w203, "PSU.xlsx" ("string")) -> (w212:string)
                n101 = local write "Heater On"(w200) -> ()
                n102 = property on="Heater Enable" class="Bool (strict)"(error in=w208, "Value"=w200) -> (error out=w207:errorcluster)  [unwired: 1 in, 1 out]
                n103 = Build Path(base path=w204, name or relative path=w215) -> (appended path=w216:path)
                n104 = Build Path(base path=w204, name or relative path=w212) -> (appended path=w211:path)
                n105 = while {
                  tunnel: w211 -> [w233]
                  tunnel: w202 -> [_]
                  tunnel: w194 -> [w229]
                  stop <- w230 stop-if-true
                  n106 = Wait Until Next ms Multiple(millisecond multiple=w229) -> ()  [unwired: 1 out]
                  n107 = local read "Heater Logging"() -> (w235:bool)
                  n108 = local read "Heater Monitor"() -> (w232:waveform(dbl)[])
                  n109 = local read "PSU_Monitor"() -> (w231:waveform(dbl)[])
                  n110 = Not(x=w235) -> (.not. x?=w230:bool)
                  n111 = Merge Signals(w232, w231) -> (w234:dynamicdata)
                  n112 = call "Write Voltage and Current Log File"("Signals"=w234, "Flush? (T)"=w230, "Filename"=w233) -> ()  [unwired: 14 in, 3 out]
                }
                n113 = while {
                  tunnel: w216 -> [w228]
                  tunnel: w202 -> [_]
                  tunnel: w193 -> [w222]
                  stop <- w226 stop-if-true
                  n114 = local read "Heater Logging"() -> (w223:bool)
                  n115 = local read "TLUP_Temperatures"() -> (w224:waveform(dbl)[])
                  n116 = local read "TVC_Temperatures"() -> (w225:waveform(dbl)[])
                  n117 = Wait Until Next ms Multiple(millisecond multiple=w222) -> ()  [unwired: 1 out]
                  n118 = Not(x=w223) -> (.not. x?=w226:bool)
                  n119 = Merge Signals(w225, w224) -> (w227:dynamicdata)
                  n120 = call "Write Temperature Log File"("Signals"=w227, "Flush? (T)"=w226, "Filename"=w228) -> ()  [unwired: 14 in, 3 out]
                }
                n121 = call "DelayTimer.vi"("Formatted \nTime Ref"=w197, "FormatString"="Heater On: %M:%S", "error in (no error)"=w207, "Delay(s)"=w190) -> ("error out"=w219:errorcluster)  [unwired: 7 in]
                n122 = property on="Heater Enable" class="Bool (strict)"(error in=w219, "Value"=w201) -> (error out=w206:errorcluster)  [unwired: 1 in, 1 out]
                n123 = local write "Heater On"(w201) -> ()
                n124 = call "DelayTimer.vi"("Formatted \nTime Ref"=w197, "FormatString"=" Post-Log: %M:%S", "error in (no error)"=w206, "Delay(s)"=w189) -> ("error out"=w205:errorcluster)  [unwired: 7 in]
                n125 = property on="Heater \nLogging" class="Bool (strict)"(error in=w205, "Value"=FALSE ("Heater Logging")) -> (error out=w217:errorcluster)  [unwired: 1 in, 1 out]
              }
              frame "Actuation Test" {
                # "Test storage Directory"
                # "TestPrefix"
                # "Actuation Test\nStart video\nExecute Python code"
                n126 = Unbundle By Name(w236) -> ("ActuationsPerLoop"=w240:i32)
                n127 = property on="Status" class="Str"(error in=w248, "Value"="Actuation Test" ("Status")) -> (error out=w244:errorcluster)  [unwired: 1 in, 1 out]
                n128 = Unbundle By Name(w239) -> ("Pre-Log (s)"=w238:dbl, "Post-Log(s)"=w237:dbl)
                n129 = for {
                  N: w240 -> [_]
                  shift-right: [w254] -> w246
                  shift-left: w244 -> [w259]
                  tunnel: w242 -> [w269]
                  tunnel: w245 -> [w279]
                  tunnel: w245 -> [w274]
                  tunnel: w245 -> [w272]
                  tunnel: "Video" ("string") -> [w267]
                  tunnel: w241 -> [w263]
                  tunnel: w241 -> [w262]
                  tunnel: w238 -> [w253]
                  tunnel: w237 -> [w252]
                  tunnel: w236 -> [w249]
                  i -> [w281]
                  stop <- w254 stop-if-true
                  # "Add Actuation\nto TestPrefix"
                  # "call Python script"
                  n130 = Format Into String(format string="A%d_", initial string=w269, w281) -> (resulting string=w268:string)  [unwired: 1 in, 1 out]
                  n131 = property on="Actuation\n Logging" class="Bool (strict)"(error in=w259, "Value"=TRUE ("Actuation Logging")) -> (error out=w260:errorcluster)  [unwired: 1 in, 1 out]
                  n132 = Concatenate Strings(w268, w267) -> (w266:string)
                  n133 = local read "FFMPEG exe"() -> (w270:path)
                  n134 = local read "Camera"() -> (w271:string)
                  n135 = Unbundle By Name(w249) -> ("PSU \nLog Period (ms)"=w251:i64, "Temperature\nLog Period(ms)"=w250:i64)
                  n136 = call "StartVideoCapture.vi"("Video Camera"=w271, "Path to FFMPEG"=w270, "error in (no error)"=w260, "SaveFile"=w266, "Output Directory"=w272) -> ("error out"=w261:errorcluster, "FFMpegProcess"=w265:T9)  [unwired: 5 in]
                  n137 = Concatenate Strings(w268, "PSU.xlsx" ("string")) -> (w277:string)
                  n138 = Build Path(base path=w274, name or relative path=w277) -> (appended path=w276:path)
                  n139 = local read "Path to Actuation Script"() -> (w273:path)
                  n140 = Concatenate Strings(w268, "Temp.xlsx" ("string")) -> (w280:string)
                  n141 = call "DelayTimer.vi"("Formatted \nTime Ref"=w263, "FormatString"="Pre-Log: %M:%S", "error in (no error)"=w261, "Delay(s)"=w253) -> ("error out"=w275:errorcluster)  [unwired: 7 in]
                  n142 = Build Path(base path=w279, name or relative path=w280) -> (appended path=w278:path)
                  n143 = while {
                    tunnel: w278 -> [w298]
                    tunnel: w261 -> [_]
                    tunnel: w250 -> [w292]
                    stop <- w296 stop-if-true
                    # "write log file, \nbuffer to memory\nflush on exit"
                    # "write Temperature log"
                    n144 = Wait Until Next ms Multiple(millisecond multiple=w292) -> ()  [unwired: 1 out]
                    n145 = local read "TLUP_Temperatures"() -> (w293:waveform(dbl)[])
                    n146 = local read "Actuation Logging"() -> (w295:bool)
                    n147 = local read "TVC_Temperatures"() -> (w294:waveform(dbl)[])
                    n148 = Not(x=w295) -> (.not. x?=w296:bool)
                    n149 = Merge Signals(w294, w293) -> (w297:dynamicdata)
                    n150 = call "Write Actuation Temperature Log"("Signals"=w297, "Flush? (T)"=w296, "Filename"=w298) -> ()  [unwired: 14 in, 3 out]
                  }
                  n151 = call "RunPythonCode.vi"("Path to Actuation Script"=w273, "COM Port"="COM Port", "error in (no error)"=w275, "TestPrefix"=w268, "Output base directory"=w272) -> ("error out"=w255:errorcluster)  [unwired: 5 in, 1 out]
                  n152 = while {
                    tunnel: w276 -> [w302]
                    tunnel: w261 -> [_]
                    tunnel: w251 -> [w299]
                    stop <- w300 stop-if-true
                    # "write log file, \nbuffer to memory\nflush on exit"
                    # "write Board PSU log"
                    n153 = local read "Actuation Logging"() -> (w301:bool)
                    n154 = Wait Until Next ms Multiple(millisecond multiple=w299) -> ()  [unwired: 1 out]
                    n155 = local read "PSU_Monitor"() -> (w303:waveform(dbl)[])
                    n156 = Not(x=w301) -> (.not. x?=w300:bool)
                    n157 = call "Write Actuation PSU Log"("Signals"=w303, "Flush? (T)"=w300, "Filename"=w302) -> ()  [unwired: 14 in, 3 out]
                  }
                  n158 = flat-sequence {
                    tunnel: w265 -> [w291]
                    tunnel: w262 -> [w290]
                    tunnel: w255 -> [w285]
                    tunnel: [w285] -> w254
                    tunnel: w252 -> [w284]
                    frame #0 {
                      n159 = call "DelayTimer.vi"("Formatted \nTime Ref"=w290, "FormatString"="Post-Log: %M:%S", "Delay(s)"=w284) -> ("error out"=w289:errorcluster)  [unwired: 8 in]
                      n160 = call "Stop FFMpeg Process.vi"("error in (no error)"=w289, "FFMpegProcess"=w291) -> ("error out"=w286:errorcluster)  [unwired: 9 in]
                      n161 = property on="Actuation\n Logging" class="Bool (strict)"(error in=w286, "Value"=FALSE ("Actuation Logging")) -> ()  [unwired: 1 in, 2 out]
                    }
                  }
                }
              }
            }
          }
          n162 = Equal To 0?(x="CyclesRemaining") -> (x = 0?=w158:bool)
          n163 = Select(t=TestExecStates."AbortExit", s=w152, f=TestExecStates."Shutdown" ("State")) -> (s? t:f=w154:T4)
          n164 = Or(x=w158, y=w152) -> (x .or. y?=w157:bool)
        }
      }
      frame "Shutdown" {
        w325 = FALSE ("PSU Enable")
        # "stop all logging and make sure power supplies are off"
        n165 = property on="Status" class="Str"(error in=w328, "Value"="Tests Finished" ("Status")) -> (error out=w327:errorcluster)  [unwired: 1 in, 1 out]
        n166 = local write "Heater Logging"(w325) -> ()
        n167 = local write "PSU Enable"(w325) -> ()
        n168 = local write "Master Logging"(w325) -> ()
        n169 = local write "Heater Enable"(w325) -> ()
        n170 = local write "Actuation Logging"(w325) -> ()
      }
      frame "AbortExit" {
        # "Display Error message and clear errors"
        n171 = flat-sequence {
          tunnel: w331 -> [w337]
          tunnel: [w337] -> w330
          frame #0 {
            w338 = FALSE
            n172 = local write "Heater Enable"(w338) -> ()
            n173 = local write "Actuation Logging"(w338) -> ()
            n174 = local write "Master Logging"(w338) -> ()
            n175 = local write "Heater Logging"(w338) -> ()
            n176 = local write "PSU Enable"(w338) -> ()
          }
        }
        n177 = call <vilib>:"Simple Error Handler.vi"("error in (no error)"=w330) -> ("error out"=w333:errorcluster)  [unwired: 4 in, 4 out]
        n178 = call <vilib>:"Clear Errors.vi"("error in (no error)"=w333) -> ("error out"=w332:errorcluster)  [unwired: 5 in, 1 out]
        n179 = property on="Status" class="Str"(error in=w332, "Value"="Abort error Triggered" ("Status")) -> (error out=w335:errorcluster)  [unwired: 1 in, 1 out]
      }
    }
  }
  n180 = property on="Master Logging" class="Bool (strict)"("Value"=FALSE ("Master Logging")) -> (error out=w3:errorcluster)  [unwired: 2 in, 1 out]
  n181 = while {
    tunnel: [w339] -> w1
    tunnel: w3 -> [_]
    stop <- w339 stop-if-true
    # "Wait until master logging goes true"
    n182 = local read "Master Logging"() -> (w339:bool)
    n183 = Wait Until Next ms Multiple(millisecond multiple=u32 100) -> ()  [unwired: 1 out]
  }
  n184 = case shown="True" w1 {
    frame False {
    }
    frame True {
      n185 = local read "TestDefinition"() -> (w342:T2)
      n186 = Unbundle By Name(w342) -> ("Temperature\nLog Period(ms)"=w343:i64)
      n187 = while {
        tunnel: w343 -> [w357]
        stop <- w360 continue-if-true
        # "draw graph of  Temperatures"
        n188 = local read "TLUP_Temperatures"() -> (w358:waveform(dbl)[])
        n189 = local read "TVC_Temperatures"() -> (w354:waveform(dbl)[])
        n190 = Wait Until Next ms Multiple(millisecond multiple=w357) -> ()  [unwired: 1 out]
        n191 = local read "ControlChannel"() -> (w352:u16)
        n192 = Merge Signals(w354, w358) -> (→"Temperatures":dynamicdata)
        n193 = Index Array(array=w354, index=w352) -> (element=w355:waveform(dbl))
        n194 = local read "Master Logging"() -> (w360:bool)
        n195 = Unbundle By Name(w355) -> ("Y"=w356:dbl[])
        n196 = Index Array(array=w356) -> (element=→"Trigger Point Reading":dbl)  [unwired: 1 in]
      }
      n197 = local read "TopFolderPrefix"() -> (w346:string)
      n198 = local read "TopFolderPath"() -> (w347:path)
      n199 = Concatenate Strings(w346, "_Temp.xlsx") -> (w351:string)
      n200 = Build Path(base path=w347, name or relative path=w351) -> (appended path=w350:path)
      n201 = while {
        tunnel: w350 -> [w372]
        tunnel: w343 -> [w366]
        i -> [w364]
        stop <- w370 stop-if-true
        # "write Temperature log\nwrite log file, buffer to memory\nflush on exit or every 100 readings"
        n202 = local read "Master Logging"() -> (w369:bool)
        n203 = Wait Until Next ms Multiple(millisecond multiple=w366) -> ()  [unwired: 1 out]
        n204 = local read "TLUP_Temperatures"() -> (w367:waveform(dbl)[])
        n205 = local read "TVC_Temperatures"() -> (w368:waveform(dbl)[])
        n206 = Quotient & Remainder(x=w364, y=100) -> (x-y*floor(x/y)=w362:i32)  [unwired: 1 out]
        n207 = Not(x=w369) -> (.not. x?=w370:bool)
        n208 = Equal To 0?(x=w362) -> (x = 0?=w361:bool)
        n209 = Or(x=w370, y=w361) -> (x .or. y?=w365:bool)
        n210 = Merge Signals(w368, w367) -> (w371:dynamicdata)
        n211 = call "Write Master Temperature"("Signals"=w371, "Flush? (T)"=w365, "Filename"=w372) -> ()  [unwired: 14 in, 3 out]
      }
      n212 = Unbundle By Name(w342) -> ("PSU \nLog Period (ms)"=w341:i64)
      n213 = Concatenate Strings(w346, "_PSU.xlsx") -> (w349:string)
      n214 = Build Path(base path=w347, name or relative path=w349) -> (appended path=w348:path)
      n215 = while {
        tunnel: w348 -> [w383]
        tunnel: w341 -> [w381]
        i -> [w374]
        stop <- w375 stop-if-true
        # "write Board PSU log\nwrite log file, buffer to memory\nflush on exit or every 100 readings"
        n216 = Wait Until Next ms Multiple(millisecond multiple=w381) -> ()  [unwired: 1 out]
        n217 = local read "Master Logging"() -> (w382:bool)
        n218 = local read "Heater Monitor"() -> (w379:waveform(dbl)[])
        n219 = local read "PSU_Monitor"() -> (w384:waveform(dbl)[])
        n220 = Quotient & Remainder(x=w374, y=1000) -> (x-y*floor(x/y)=w377:i32)  [unwired: 1 out]
        n221 = Not(x=w382) -> (.not. x?=w375:bool)
        n222 = Equal To 0?(x=w377) -> (x = 0?=w378:bool)
        n223 = Merge Signals(w379, w384) -> (w380:dynamicdata)
        n224 = Or(x=w375, y=w378) -> (x .or. y?=w373:bool)
        n225 = call "Write Master PSU Log"("Signals"=w380, "Flush? (T)"=w373, "Filename"=w383) -> ()  [unwired: 14 in, 3 out]
      }
    }
  }
